vi "VIUnit - VI Tree.vi"() -> ()   [LabVIEW 2013]
uses:
  Classes/TestResult/TestResult.lvclass
  Classes/TestCase/TestCase.lvclass
  Classes/TestSuite/TestSuite.lvclass
  Classes/_TextTestResult/_TextTestResult.lvclass
  Classes/TextTestRunner/TextTestRunner.lvclass
  Classes/TestLoader/TestLoader.lvclass
  Templates/TestCase/TemplateTestCase.lvclass
  Templates/TestSuite/TemplateTestSuite.lvclass
  <userlib>/_OpenG.lib/comparison/comparison.llb/String Changed__ogtk.vi
  User Interfaces/Graphical Test Runner/Graphical Test Runner Support/GraphicalTestRunner.lvlib
  Programmatic API/VI Tester API.lvlib
  Libraries/VITesterUtilities.lvlib
panel:
  in  "Boolean":bool
  # "JKI VI Tester for LabVIEW\nhttp://jki.net/vi-tester\nCopyright (C) 2007-2019, JKI <info@jki.net>\nALL RIGHTS RESERVED"
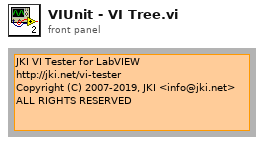
[diagram p1: front panel]
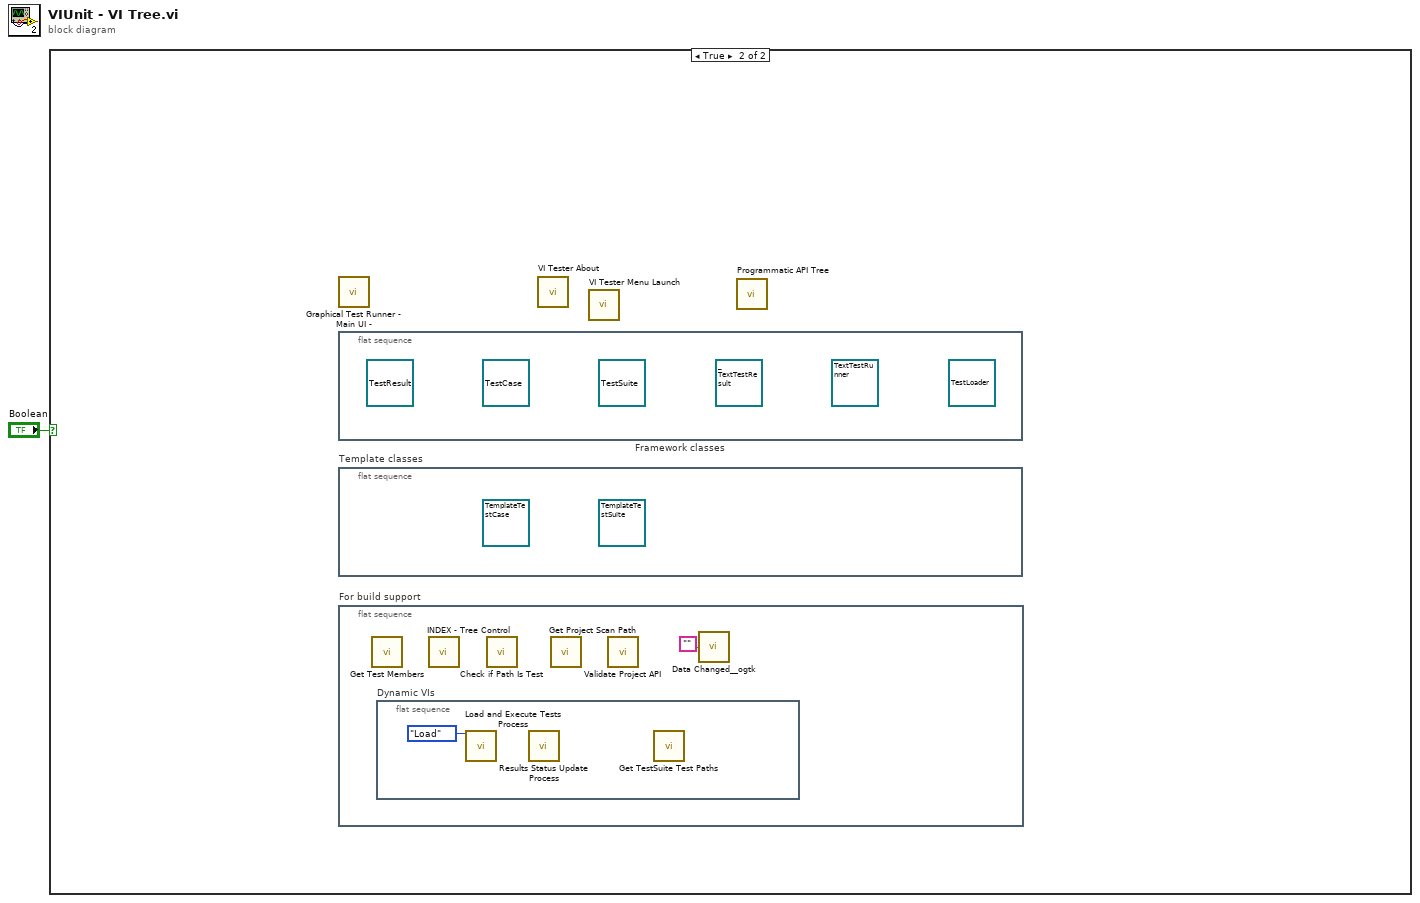
[diagram p0: block diagram]
diagram:
  n1 = case shown="True" "Boolean" {
    frame False {
    }
    frame True {
      n2 = call "Graphical Test Runner - Main UI - .vi"() -> ()  [unwired: 12 in]
      n3 = flat-sequence "Framework classes" {
        frame #0 {
          (unwired) refnum<class "TestLoader.lvclass"> refnum ("TestLoader.lvclass")
          (unwired) refnum<class "TextTestRunner.lvclass"> refnum ("TextTestRunner.lvclass")
          (unwired) refnum<class "_TextTestResult.lvclass"> refnum ("_TextTestResult.lvclass")
          (unwired) refnum<class "TestSuite.lvclass"> refnum ("TestSuite.lvclass")
          (unwired) refnum<class "TestCase.lvclass"> refnum ("TestCase.lvclass")
          (unwired) refnum<class "TestResult.lvclass"> refnum ("TestResult.lvclass")
        }
      }
      n4 = flat-sequence "Template classes" {
        frame #0 {
          (unwired) refnum<class "TemplateTestSuite.lvclass"> refnum ("TemplateTestSuite.lvclass")
          (unwired) refnum<class "TemplateTestCase.lvclass"> refnum ("TemplateTestCase.lvclass")
        }
      }
      n5 = flat-sequence "For build support" {
        frame #0 {
          n6 = call "Get Test Members.vi"() -> ()  [unwired: 10 in, 2 out]
          n7 = flat-sequence "Dynamic VIs" {
            frame #0 {
              n8 = call "Load and Execute Tests Process.vi"("Operation"=enum16{"Load", "Run Test", "Run All Tests"}."Load") -> ()  [unwired: 13 in, 2 out]
              n9 = call "Results Status Update Process.vi"() -> ()  [unwired: 11 in, 1 out]
              n10 = call "Get TestSuite Test Paths.vi"() -> ()  [unwired: 10 in, 2 out]
            }
          }
          n11 = call "INDEX - Tree Control.vi"() -> ()  [unwired: 1 in]
          n12 = call "Check if Path Is Test.vi"() -> ()  [unwired: 11 in, 1 out]
          n13 = call "Get Project Scan Path.vi"() -> ()  [unwired: 9 in, 3 out]
          n14 = call "Validate Project API.vi"() -> ()  [unwired: 1 in]
          n15 = call-poly <userlib>:"Data Changed__ogtk.vi"("String"="") -> ()  [unwired: 1 out]
        }
      }
      n16 = call "VI Tester About.vi"() -> ()  [unwired: 1 in]
      n17 = call "VI Tester Menu Launch.vi"() -> ()  [unwired: 1 in]
      n18 = call "Programmatic API Tree.vi"() -> ()  [unwired: 1 in]
    }
  }
